vi "Open.vi"(8 "error in (no error)":errorcluster, 10 "exe path":path, 11 "LT_UpgradeFlash in":refnum<class "LT_UpgradeFlash.lvclass">) -> (0 "error out":errorcluster, 1 "resultStr":string, 2 "ActionResult":bool, 3 "LT_UpgradeFlash out":refnum<class "LT_UpgradeFlash.lvclass">)   [LabVIEW 2017, in "LT_UpgradeFlash.lvclass"]
uses:
  LT_UpgradeFlash.lvclass
  D:/Project/Tymphany/LT_UpgradeFlash/New_Lib/LT_UpgradeFlash_dll/LT_UpgradeFlash_dll/bin/Debug/LT_UpgradeFlash_dll.dll
  New_Lib/LT_UpgradeFlash_dll/LT_UpgradeFlash_dll/bin/Debug/LT_UpgradeFlash_dll.dll
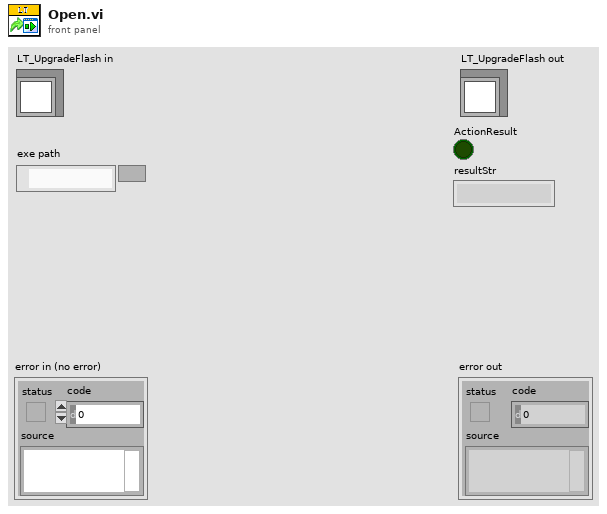
[diagram p1: front panel]
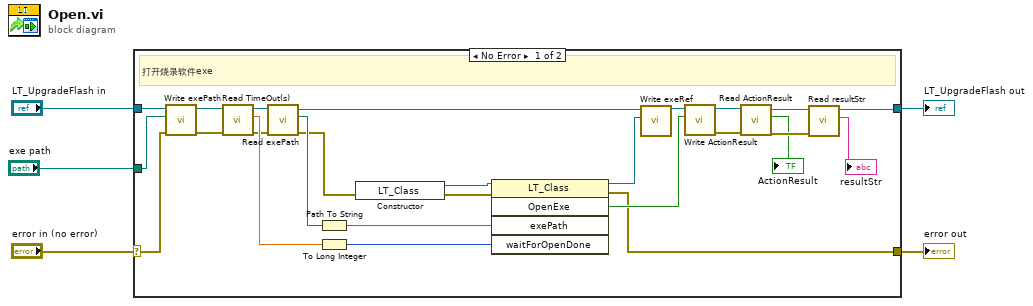
[diagram p0: block diagram]
diagram:
  n1 = case shown="No Error" "error in (no error)" {
    selector: "error in (no error)" -> [w17 w33]
    tunnel: [w22 w33] -> w4
    tunnel: [w10 w32] -> w2
    tunnel: "LT_UpgradeFlash in" -> [w21 w32]
    tunnel: "exe path" -> [w15 _]
    frame No Error {
      # "打开烧录软件exe"
      n2 = call-dynamic "Write exePath.vi"("error in (no error)"=w17, "exePath"=w15, "LT_UpgradeFlash in"=w21) -> ("error out"=w19:errorcluster, "LT_UpgradeFlash out"=w20:refnum<class "LT_UpgradeFlash.lvclass">)  [unwired: 7 in]
      n3 = call-dynamic "Read TimeOut(s).vi"("error in (no error)"=w19, "LT_UpgradeFlash in"=w20) -> ("error out"=w18:errorcluster, "TimeOut(s)"=w28:dbl, "LT_UpgradeFlash out"=w31:refnum<class "LT_UpgradeFlash.lvclass">)  [unwired: 7 in]
      n4 = call-dynamic "Read exePath.vi"("error in (no error)"=w18, "LT_UpgradeFlash in"=w31) -> ("error out"=w16:errorcluster, "exePath"=w30:path, "LT_UpgradeFlash out"=w25:refnum<class "LT_UpgradeFlash.lvclass">)  [unwired: 7 in]
      n5 = Path To String(path=w30) -> (string=w29:string)
      n6 = To Long Integer(number=w28) -> (32bit integer=w27:i32)
      n7 = constructor class="LT_Class"(error in=w16) -> (reference out=w7:refnum<k24>, error out=w23:errorcluster)  [unwired: 2 in, 1 out]
      n8 = invoke class="LT_Class" method="OpenExe"(reference=w7, error in=w23, "exePath"=w29, "waitForOpenDone"=w27) -> (reference out=w6:refnum<k24>, error out=w22:errorcluster, "OpenExe"=w26:bool)  [unwired: 1 in, 2 out]
      n9 = call-dynamic "Write exeRef.vi"("exeRef"=w6, "LT_UpgradeFlash in"=w25) -> ("LT_UpgradeFlash out"=w24:refnum<class "LT_UpgradeFlash.lvclass">)  [unwired: 8 in, 1 out]
      n10 = call-dynamic "Write ActionResult.vi"("ActionResult"=w26, "LT_UpgradeFlash in"=w24) -> ("error out"=w13:errorcluster, "LT_UpgradeFlash out"=w14:refnum<class "LT_UpgradeFlash.lvclass">)  [unwired: 8 in]
      n11 = call-dynamic "Read ActionResult.vi"("error in (no error)"=w13, "LT_UpgradeFlash in"=w14) -> ("error out"=w11:errorcluster, "ActionResult"=→"ActionResult":bool, "LT_UpgradeFlash out"=w12:refnum<class "LT_UpgradeFlash.lvclass">)  [unwired: 7 in]
      n12 = call-dynamic "Read resultStr.vi"("error in (no error)"=w11, "LT_UpgradeFlash in"=w12) -> ("resultStr"=→"resultStr":string, "LT_UpgradeFlash out"=w10:refnum<class "LT_UpgradeFlash.lvclass">)  [unwired: 7 in, 1 out]
    }
    frame Error {
    }
  }
  "error out" <- w4
  "LT_UpgradeFlash out" <- w2
